vi "EnqueueDatagram.vi"(8 "error in (no error)":errorcluster, 9 "Enqueue at Front? (F)":bool, 10 "mqttCmd":refnum<class "BaseMqttMsg.lvclass">, 11 "mqtt in":refnum<class "MQTT Client.lvclass">) -> (0 "error out":errorcluster, 3 "mqtt out":refnum<class "MQTT Client.lvclass">)   [LabVIEW 2020, in "MQTT Client.lvclass"]
uses:
  MQTT Client.lvclass
  mqttCmd/BaseMqttMsg.lvclass
  MQTT Client.lvclass/MQTT Client.ctl
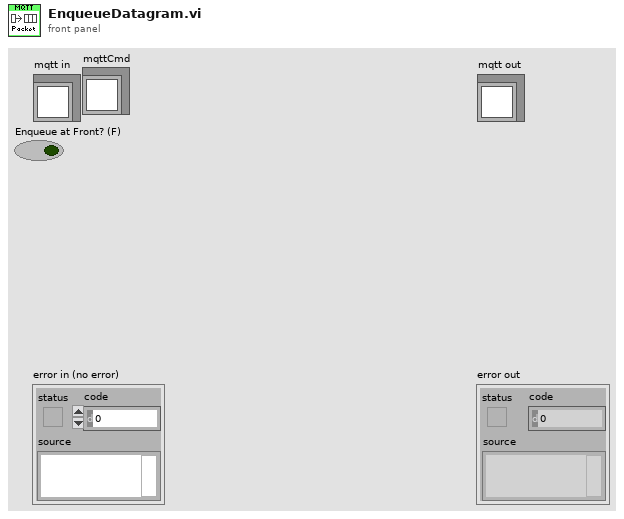
[diagram p1: front panel]
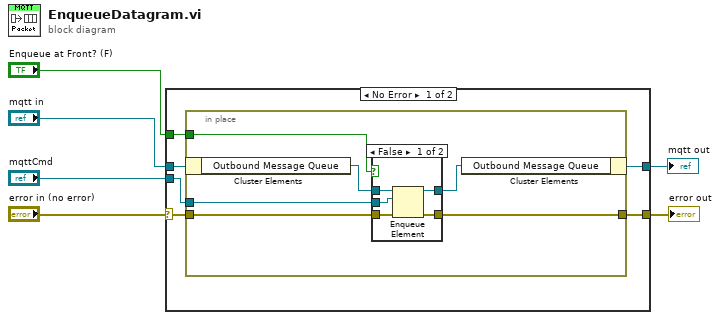
[diagram p0: block diagram]
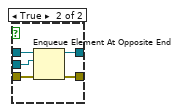
[diagram p2: hidden frame]
diagram:
  n1 = case shown="No Error" "error in (no error)" {
    selector: "error in (no error)" -> [w9 w30]
    tunnel: [w10 w30] -> w5
    tunnel: [w11 w29] -> w3
    tunnel: "mqtt in" -> [w12 w29]
    tunnel: "mqttCmd" -> [w8 _]
    tunnel: "Enqueue at Front? (F)" -> [w7 _]
    frame No Error {
      n2 = in-place {
        in-place-border: w9 -> [w16]
        in-place-border: [w15] -> w10
        in-place-border: w8 -> [w14]
        in-place-border: w7 -> [w13]
        n3 = in-place-cluster #1(w12) -> ("Outbound Message Queue"=w18:refnum<queue>)
        n4 = case shown="False" w13 {
          tunnel: w18 -> [w23 w27]
          tunnel: [w22 w26] -> w17
          tunnel: w16 -> [w21 w28]
          tunnel: [w20 w25] -> w15
          tunnel: w14 -> [w19 w24]
          frame False {
            n5 = Enqueue Element(queue=w23, element=w19, error in (no error)=w21) -> (queue out=w22:refnum<queue>, error out=w20:errorcluster)  [unwired: 1 in, 1 out]
          }
          frame True {
            n6 = Enqueue Element At Opposite End(queue=w27, element=w24, error in (no error)=w28) -> (queue out=w26:refnum<queue>, error out=w25:errorcluster)  [unwired: 1 in, 1 out]
          }
        }
        n7 = in-place-cluster #1("Outbound Message Queue"=w17) -> (w11:refnum<class "MQTT Client.lvclass">)
      }
    }
    frame Error {
    }
  }
  "error out" <- w5
  "mqtt out" <- w3
